vi "Exponential Filter with IC (final value).vi"(3 "init/cont (init:F)":bool, 4 "initial filter state":dbl format="%.2f", 5 "filter coefficients":T1 {"Forward Coefficients" format="%.2f"; "Reverse Coefficients" format="%.2f"}, 6 "X":dbl[](array[numeric]) format="%.2f") -> (0 "error":i32, 1 "final filter state":dbl format="%.2f", 2 "filtered X (final value)":dbl format="%.2f")   [LabVIEW 2017]
doc: "Applies a single time constant exponential averaging on the input signal X based on the filter coefficients, and returns only the last value of the filtered signal.\nThe initial filter state and the final filter state parameters keep track of the internal state of the filter to ensure continuous operation of the filter if continuous mode is used."
uses:
  <resource>/lvanlys.dll
panel:
  # "Exponential Filter with I.C."
  # "Returning final value ONLY"
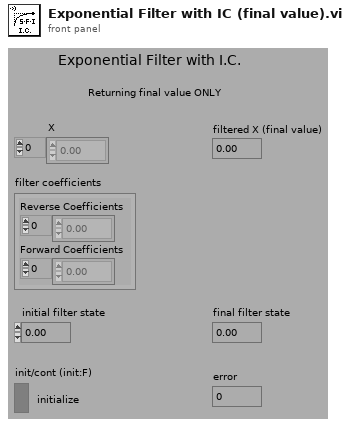
[diagram p1: front panel]
types:
  T1 = cluster{"Reverse Coefficients":dbl[], "Forward Coefficients":dbl[]}
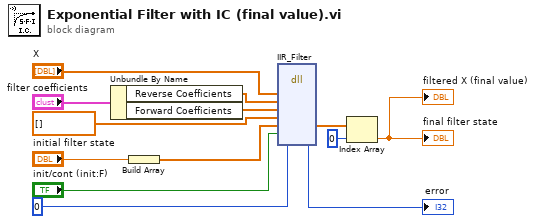
[diagram p0: block diagram]
diagram:
  n1 = Unbundle By Name("filter coefficients") -> ("Reverse Coefficients"=w8:dbl[], "Forward Coefficients"=w7:dbl[])
  n2 = Build Array("initial filter state") -> (w5:dbl[])
  n3 = dll-call lib="C:/Program Files (x86)/National Instruments/LabVIEW 2017/resource/lvanlys.*" fn="IIR_Filter"("X"="X", "Reverse Coefficients"=w8, "Forward Coefficients"=w7, "Initial X Conditions"=dbl[] [], "output param"=w5, "init/cont (init:F)"="init/cont (init:F)", "Input Value"=0) -> ("output param"=w1:dbl[], "Input Value"=→"error":i32)  [unwired: 9 in, 2 out]
  n4 = Index Array(array=w1, index=0) -> (element=→"final filter state" →"filtered X (final value)":dbl)
